vi "Find Center Setup.vi"(0 "Carrier Tray":T1, 1 "Tray Number":dbl format="%#_13g", 2 "Position":i32, 3 "Assembly Type":string) -> (7 "Assembly Tray Out":T1)   [LabVIEW 2021, in "Assembly Tray.lvclass"]
uses:
  Assembly Tray.lvclass
  Find Tray.ctl
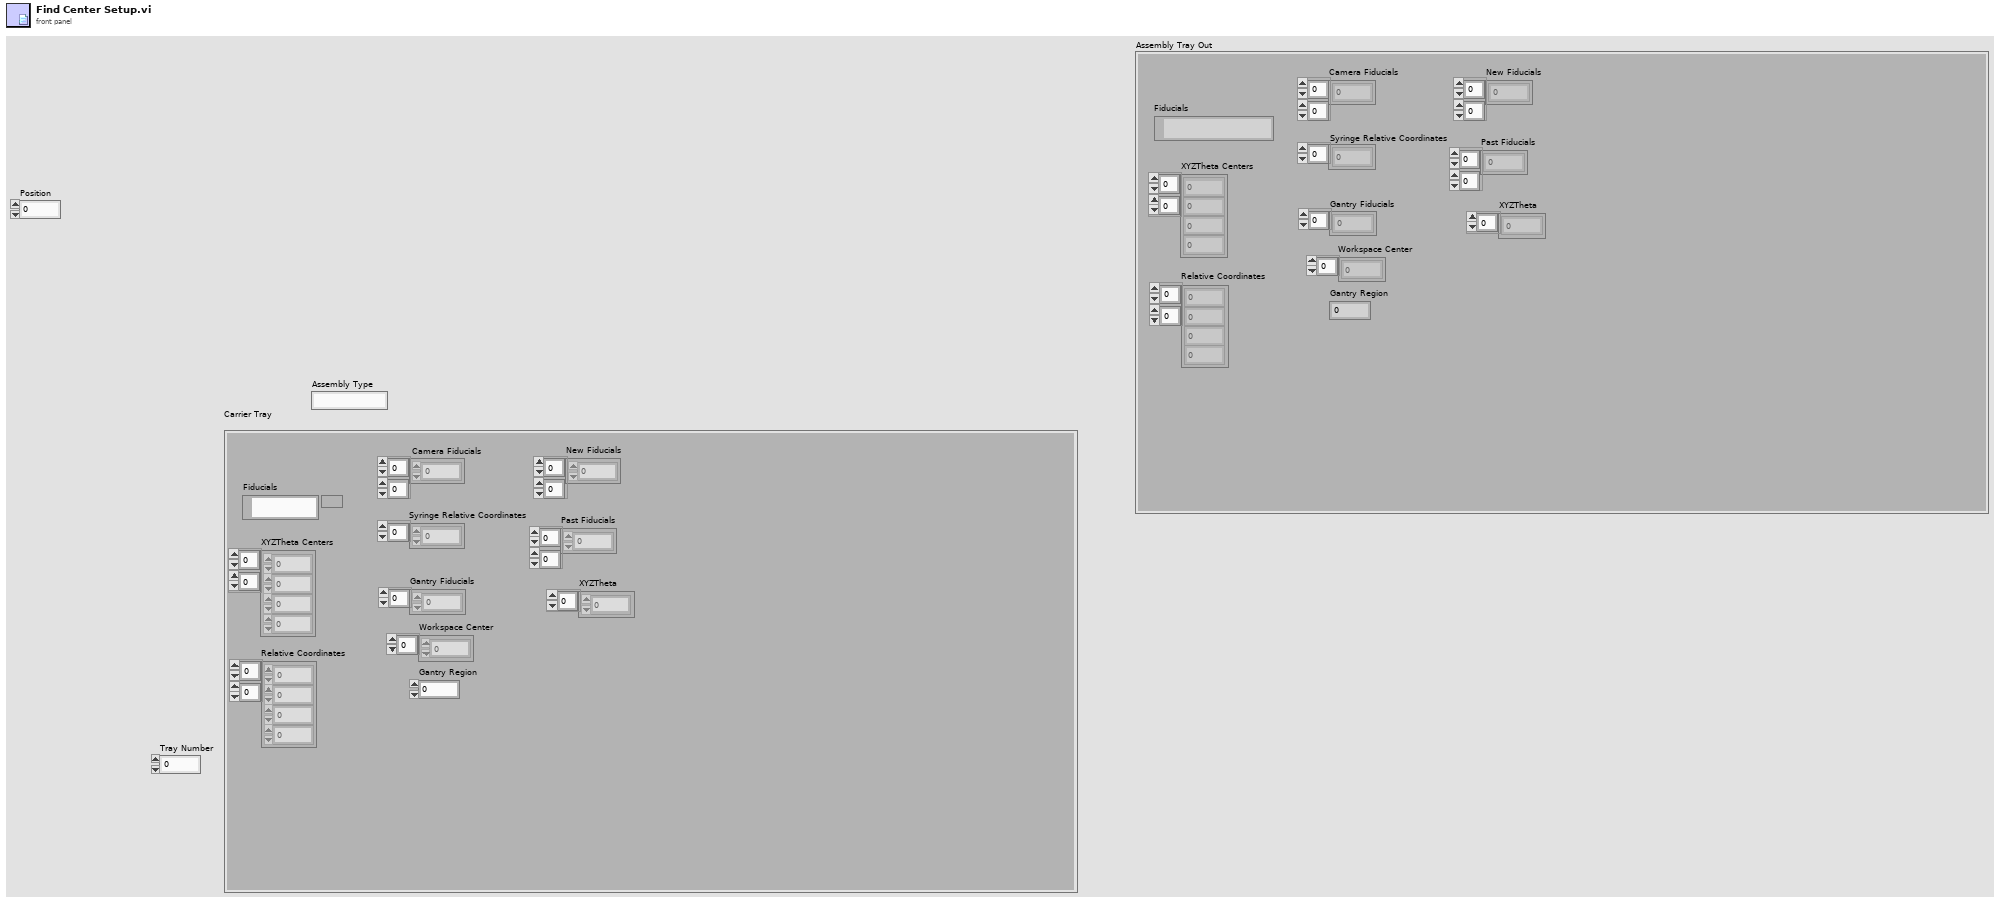
[diagram p1: front panel]
types:
  T1 = typedef "Assembly Tray.lvclass/Find Tray.ctl" = cluster{"Gantry Fiducials":dbl[], "Relative Coordinates":dbl[][], "Camera Fiducials":dbl[][], "XYZTheta Centers":dbl[][], "Workspace Center":dbl[], "Syringe Relative Coordinates":dbl[], "Gantry Region":dbl, "Fiducials":path, "New Fiducials":dbl[][], "Past Fiducials":dbl[][], "XYZTheta":dbl[]}
  T2 = typedef "File Paths.ctl" = cluster{"Glue Pattern Folder":path, "Carrier Tray Folder":path, "Pick Up Tool Fixture Folder":path, "Components Folder":path, "Bellows Tool Offset.txt":path, "Pick Up Tool Offset.txt":path, "Dispense Tip Offset.txt":path, "Log Files":path, "Gantry Assembly Map.txt":path, "Syringe and offset map.txt":path, "Controllers Folder":path, "Local dbase config":path}
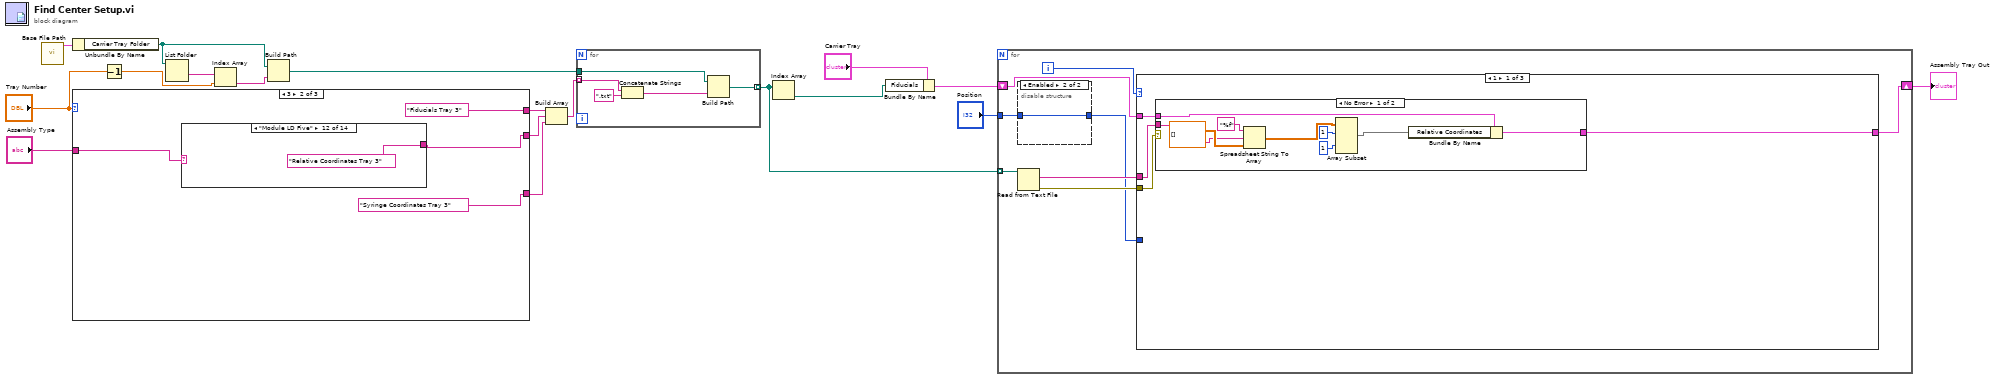
[diagram p0: block diagram]
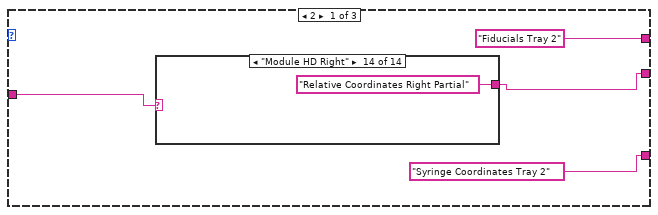
[diagram p2: hidden frame]
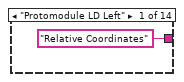
[diagram p3: hidden frame]
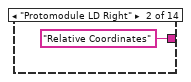
[diagram p4: hidden frame]
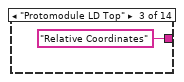
[diagram p5: hidden frame]
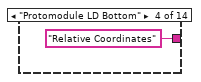
[diagram p6: hidden frame]
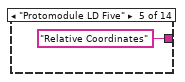
[diagram p7: hidden frame]
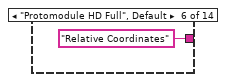
[diagram p8: hidden frame]
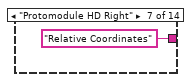
[diagram p9: hidden frame]
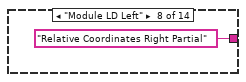
[diagram p10: hidden frame]
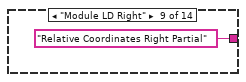
[diagram p11: hidden frame]
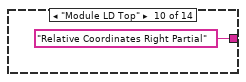
[diagram p12: hidden frame]
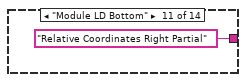
[diagram p13: hidden frame]
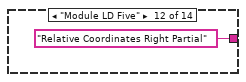
[diagram p14: hidden frame]
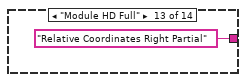
[diagram p15: hidden frame]
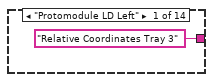
[diagram p16: hidden frame]
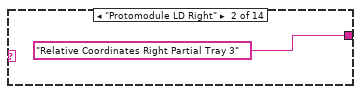
[diagram p17: hidden frame]
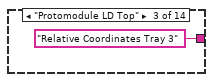
[diagram p18: hidden frame]
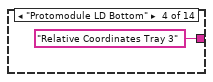
[diagram p19: hidden frame]
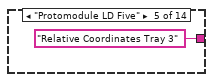
[diagram p20: hidden frame]
diagram:
  n1 = call "Base File Path.vi"() -> ("Paths Out"=w13:T2)  [unwired: 11 in]
  n2 = Unbundle By Name(w13) -> ("Carrier Tray Folder"=w6:path)
  n3 = case shown="3" "Tray Number" {
    tunnel: [w19 w37 w58] -> w9
    tunnel: "Assembly Type" -> [w20 w38 w57]
    tunnel: ["Fiducials Tray 2" ("format string") "Fiducials Tray 3" ("format string") "Fiducials" ("format string")] -> w4
    tunnel: ["Syringe Coordinates Tray 2" ("element") "Syringe Coordinates Tray 3" ("element") "Syringe Coordinates" ("element")] -> w3
    frame 2 {
      n4 = case shown="\"Module HD Right\"" w20 {
        tunnel: ["Relative Coordinates" ("format string") "Relative Coordinates" ("format string") "Relative Coordinates" ("format string") "Relative Coordinates" ("format string") "Relative Coordinates" ("format string") "Relative Coordinates" ("format string") "Relative Coordinates" ("format string") "Relative Coordinates Right Partial" ("format string") "Relative Coordinates Right Partial" ("format string") "Relative Coordinates Right Partial" ("format string") "Relative Coordinates Right Partial" ("format string") "Relative Coordinates Right Partial" ("format string") "Relative Coordinates Right Partial" ("format string") "Relative Coordinates Right Partial" ("format string")] -> w19
        frame "Protomodule LD Left" {
        }
        frame "Protomodule LD Right" {
        }
        frame "Protomodule LD Top" {
        }
        frame "Protomodule LD Bottom" {
        }
        frame "Protomodule LD Five" {
        }
        frame "Protomodule HD Full", Default {
        }
        frame "Protomodule HD Right" {
        }
        frame "Module LD Left" {
        }
        frame "Module LD Right" {
        }
        frame "Module LD Top" {
        }
        frame "Module LD Bottom" {
        }
        frame "Module LD Five" {
        }
        frame "Module HD Full" {
        }
        frame "Module HD Right" {
        }
      }
    }
    frame 3 {
      n5 = case shown="\"Module LD Five\"" w38 {
        tunnel: ["Relative Coordinates Tray 3" ("format string") "Relative Coordinates Right Partial Tray 3" ("format string") "Relative Coordinates Tray 3" ("format string") "Relative Coordinates Tray 3" ("format string") "Relative Coordinates Tray 3" ("format string") "Relative Coordinates Tray 3" ("format string") "Relative Coordinates Tray 3" ("format string") "Relative Coordinates Tray 3" ("format string") "Relative Coordinates Tray 3" ("format string") "Relative Coordinates Tray 3" ("format string") "Relative Coordinates Tray 3" ("format string") "Relative Coordinates Tray 3" ("format string") "Relative Coordinates Tray 3" ("format string") "Relative Coordinates Right Partial Tray 3" ("format string")] -> w37
        frame "Protomodule LD Left" {
        }
        frame "Protomodule LD Right" {
        }
        frame "Protomodule LD Top" {
        }
        frame "Protomodule LD Bottom" {
        }
        frame "Protomodule LD Five" {
        }
        frame "Protomodule HD Full", Default {
        }
        frame "Protomodule HD Right" {
        }
        frame "Module LD Left" {
        }
        frame "Module LD Right" {
        }
        frame "Module LD Top" {
        }
        frame "Module LD Bottom" {
        }
        frame "Module LD Five" {
        }
        frame "Module HD Full" {
        }
        frame "Module HD Right" {
        }
      }
    }
    frame 1, Default {
      n6 = case shown="\"Module HD Right\"" w57 {
        tunnel: ["Relative Coordinates" ("format string") "Relative Coordinates" ("format string") "Relative Coordinates" ("format string") "Relative Coordinates" ("format string") "Relative Coordinates" ("format string") "Relative Coordinates" ("format string") "Relative Coordinates" ("format string") "Relative Coordinates Right Partial" ("format string") "Relative Coordinates Right Partial" ("format string") "Relative Coordinates Right Partial" ("format string") "Relative Coordinates Right Partial" ("format string") "Relative Coordinates Right Partial" ("format string") "Relative Coordinates Right Partial" ("format string") "Relative Coordinates Right Partial" ("format string")] -> w58
        frame "Protomodule LD Left" {
        }
        frame "Protomodule LD Right" {
        }
        frame "Protomodule LD Top" {
        }
        frame "Protomodule LD Bottom" {
        }
        frame "Protomodule LD Five" {
        }
        frame "Protomodule HD Full", Default {
        }
        frame "Protomodule HD Right" {
        }
        frame "Module LD Left" {
        }
        frame "Module LD Right" {
        }
        frame "Module LD Top" {
        }
        frame "Module LD Bottom" {
        }
        frame "Module LD Five" {
        }
        frame "Module HD Full" {
        }
        frame "Module HD Right" {
        }
      }
    }
  }
  n7 = Decrement(x="Tray Number") -> (x-1=w11:dbl)
  n8 = List Folder(path=w6) -> (folder names=w15:string[])  [unwired: 3 in, 3 out]
  n9 = Index Array "Index Array"(array=w15, index=w11) -> (element=w14:string)
  n10 = Build Path(base path=w6, name or relative path=w14) -> (appended path=w7:path)
  n11 = Build Array(w4, w9, w3) -> (w16:string[])
  n12 = for {
    tunnel: w16 -> [w76] mode=indexing
    tunnel: w7 -> [w77]
    tunnel: [w73] -> w8 mode=indexing
    n13 = Concatenate Strings "Concatenate Strings"(w76, ".txt" ("string")) -> (w74:string)
    n14 = Build Path(base path=w77, name or relative path=w74) -> (appended path=w73:path)
  }
  n15 = Index Array "Index Array"(array=w8) -> (element=w17:path)  [unwired: 1 in]
  n16 = Bundle By Name "Bundle By Name"(cluster="Carrier Tray", "Fiducials"=w17) -> (w18:T1)
  n17 = for {
    tunnel: w8 -> [w84] mode=indexing
    shift-right: [w80] -> w12
    shift-left: w18 -> [w81]
    tunnel: "Position" -> [w79]
    i -> [w82]
    n18 = disable-structure shown="Enabled" {
      disable-tunnel: w79 -> [w87 w89]
      disable-tunnel: [w86 w89] -> w78
      frame Disabled {
        n19 = Add(x=1, y=w87) -> (x+y=w86:i32)
      }
      frame Enabled {
      }
    }
    n20 = Read from Text File(file (use dialog)=w84) -> (text=w85:string, error out=w83:errorcluster)  [unwired: 3 in, 2 out]
    n21 = case shown="1" w82 {
      tunnel: w85 -> [w92 w107 w123]
      tunnel: w83 -> [w93 w108 w122]
      tunnel: w81 -> [w91 w109 w121]
      tunnel: [w90 w106 w120] -> w80
      tunnel: w78 -> [_ _ w119]
      frame 1 {
        n22 = case shown="No Error" w93 {
          tunnel: w92 -> [w100 _]
          tunnel: [w98 w103] -> w90
          tunnel: w91 -> [w99 w103]
          frame No Error {
            n23 = Spreadsheet String To Array(format string="%f", spreadsheet string=w100, array type (2D Dbl)=dbl[][] []) -> (array=w97:dbl[][])  [unwired: 1 in]
            n24 = Array Subset(array=w97, index (row)=1 ("length"), index (col)=1 ("index (row)")) -> (w96:dbl[][])  [unwired: 2 in]
            n25 = Bundle By Name(cluster=w99, "Relative Coordinates"=w96) -> (w98:T1)
          }
          frame Error {
            n26 = One Button Dialog(message="Relative Coordinates Not Found") -> (true=w104:bool)  [unwired: 1 in]
            n27 = Stop(stop? (T)=w104) -> ()
          }
        }
      }
      frame 2 {
        n28 = case shown="No Error" w108 {
          tunnel: w107 -> [w113 _]
          tunnel: [w111 w116] -> w106
          tunnel: w109 -> [w112 w116]
          frame No Error {
            n29 = Spreadsheet String To Array(format string="%f", spreadsheet string=w113, array type (2D Dbl)=dbl[] []) -> (array=w110:dbl[])  [unwired: 1 in]
            n30 = Bundle By Name(cluster=w112, "Syringe Relative Coordinates"=w110) -> (w111:T1)
          }
          frame Error {
            n31 = One Button Dialog(message="Syringe Coordinates Not Found") -> (true=w117:bool)  [unwired: 1 in]
            n32 = Stop(stop? (T)=w117) -> ()
          }
        }
      }
      frame 0, Default {
        n33 = case shown="Error" w122 {
          tunnel: w123 -> [w129 _]
          tunnel: w121 -> [w127 w140]
          tunnel: [w128 w140] -> w120
          tunnel: w119 -> [w124 _]
          frame No Error {
            # "Commented out this Index Array Initially\nRe-enabled it to go back to original version\nAsk Jessica why she doesn't have it"
            # "Changed from Gantry Fiducials\nto Relative Fiducials to match Jessica's \ncode - 02.22.2023"
            n34 = Spreadsheet String To Array(format string="%f", spreadsheet string=w129) -> (array=w125:dbl[][])  [unwired: 2 in]
            n35 = disable-structure shown="Enabled" {
              disable-tunnel: [w135 w136] -> w126
              disable-tunnel: w125 -> [w134 w139]
              disable-tunnel: w124 -> [w131 _]
              frame Enabled {
                n36 = Index Array "Index Array"(array=w134, index (row)=w131) -> (element=w133:dbl[])  [unwired: 1 in]
                n37 = Reshape Array "Reshape Array"(w133, 6 ("dimension size")) -> (w135:dbl[])
              }
              frame Disabled {
                n38 = Delete From Array "Delete From Array"() -> ()  [unwired: 3 in, 2 out]
                n39 = Reshape Array "Reshape Array"(w139, 1 ("dimension size"), 1 ("dimension size")) -> (w136:dbl[][])
              }
            }
            n40 = Bundle By Name "Bundle By Name"(cluster=w127, "Gantry Fiducials"=w126) -> (w128:T1)
          }
          frame Error {
            n41 = One Button Dialog(message="Fiducial Data Not Found\nFind Fiducials Manually") -> ()  [unwired: 1 in, 1 out]
          }
        }
      }
    }
  }
  "Assembly Tray Out" <- w12
